vi "Display Info.vi"(7 "Layout ref":refnum<vi>, 8 "error in (no error)":errorcluster, 9 "Modify (F) /Add [T]":bool, 10 "Names in use":string[](array[string])=["PB", "Feet"], 11 "PTS-via-PB in":refnum<class "PTS-via-PB.lvclass">) -> (0 "error out":errorcluster, 1 "Names in use out":string[](array[string]), 2 "Changes Made?":bool, 3 "PTS-via-PB out":refnum<class "PTS-via-PB.lvclass">)   [LabVIEW 2013, in "PTS-via-PB.lvclass"]
uses:
  PTS-via-PB.lvclass
  ColumnVIs/Column/Column.lvclass
  TypeDefs/ColumnAppearCluster.ctl
panel:
  in  "Freq Col":T1={"Column Name"="RF Freq.", "Width"=30, "Bkgd"=[16448250], "Text"=[0]}
  in  "Name":string="PTS"
  in  "Device Description":string
  in  "SpinAPI Path":path=path "C:/SpinCore/SpinAPI/dll/spinapi.dll"
  in  "Board Num.":i32=1 max=256 step=1
  in  "Trig.\nLine":i32=23 max=256 step=1
  in  "Cancel":bool
  in  "Done":bool
  out "Names in use out":string[](array[string])
  out "Cols":refnum<class "Column.lvclass">[](array[class])
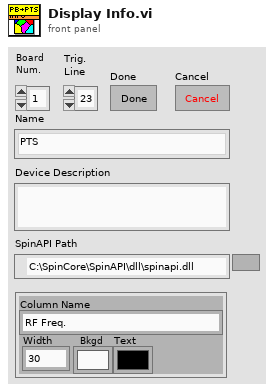
[diagram p1: front panel]
types:
  T1 = typedef "ColumnAppearCluster.ctl" = cluster{"Column Name":string, "Width":u32, "Bkgd":u32[], "Text":u32[]}
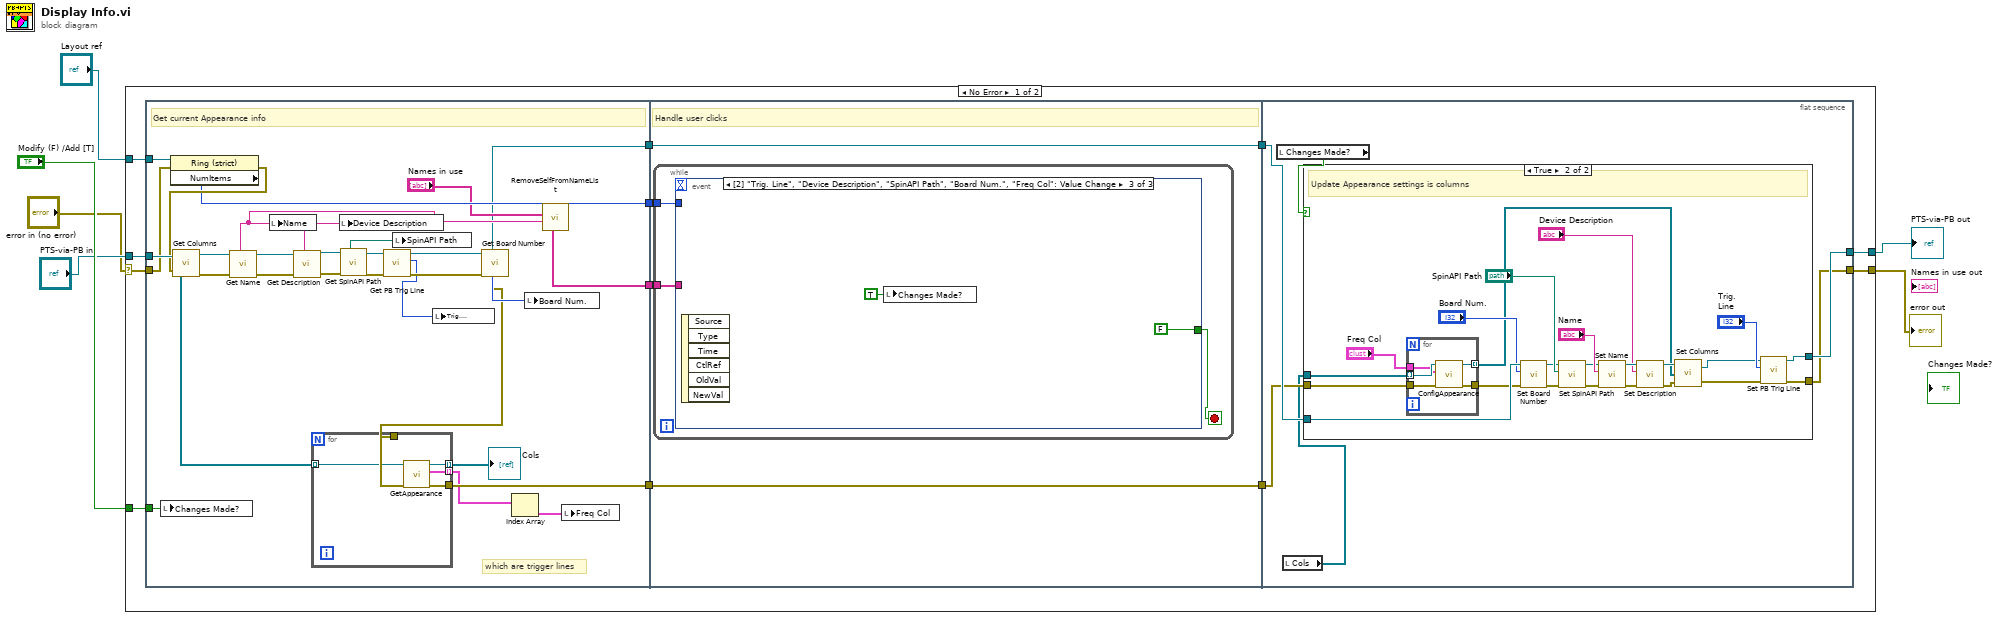
[diagram p0: block diagram]
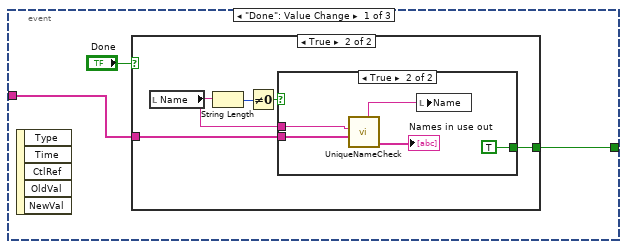
[diagram p2: hidden frame]
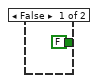
[diagram p3: hidden frame]
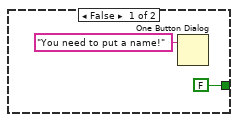
[diagram p4: hidden frame]
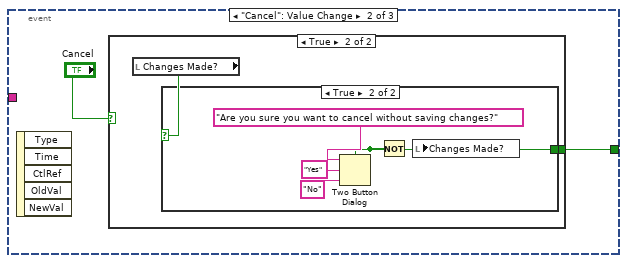
[diagram p5: hidden frame]
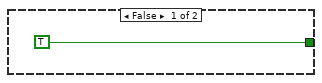
[diagram p7: hidden frame]
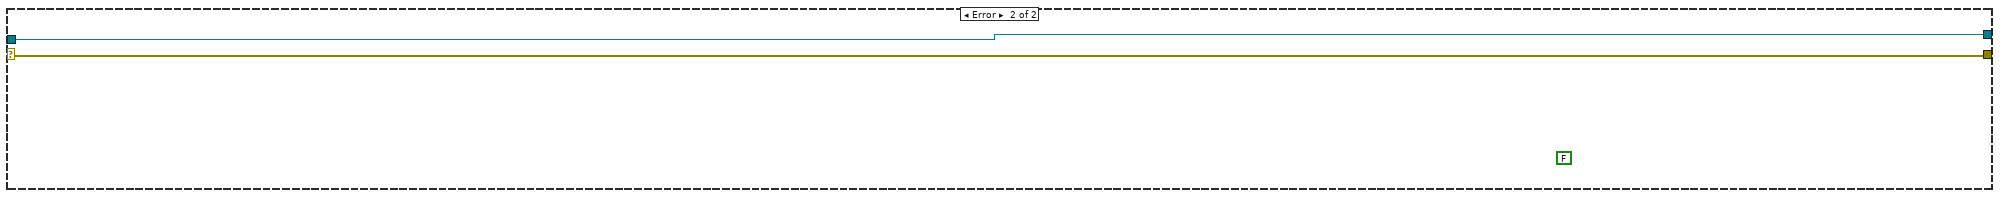
[diagram p9: hidden frame]
diagram:
  n1 = case shown="No Error" "error in (no error)" {
    selector: "error in (no error)" -> [w11 w126]
    tunnel: [w13 w127] -> w2
    tunnel: "PTS-via-PB in" -> [w18 w127]
    tunnel: [w12 w126] -> w1
    tunnel: "Layout ref" -> [w10 _]
    tunnel: "Modify (F) /Add [T]" -> [w8 _]
    frame No Error {
      n2 = flat-sequence {
        tunnel: w18 -> [w46]
        tunnel: [w19] -> w17
        tunnel: [w42] -> w15
        tunnel: w11 -> [w39]
        tunnel: w10 -> [w40]
        tunnel: [w37] -> w9
        tunnel: w8 -> [w36]
        tunnel: [w34] -> w7
        tunnel: w17 -> [w57]
        tunnel: [w57] -> w16
        tunnel: w15 -> [w56]
        tunnel: [w56] -> w14
        tunnel: w9 -> [w55]
        tunnel: w7 -> [w54]
        tunnel: w16 -> [w94]
        tunnel: w14 -> [w91]
        tunnel: [w93] -> w13
        tunnel: [w92] -> w12
        frame #0 {
          # "which are trigger lines"
          # "Get current Appearance info"
          n3 = local write "Changes Made?"(w36) -> ()
          n4 = property class="Ring (strict)"(reference=w40, error in=w39) -> (error out=w38:errorcluster, "NumItems"=w37:u32)  [unwired: 1 out]
          n5 = call-dynamic "Get Columns.vi"("Device in"=w46, "error in (no error)"=w38) -> ("Device out"=w44:refnum<class "PTS-via-PB.lvclass">, "Columns"=w29:refnum<class "Column.lvclass">[], "error out"=w43:errorcluster)
          n6 = call-dynamic "Get Name.vi"("error in (no error)"=w43, "Device in"=w44) -> ("error out"=w45:errorcluster, "Name"=w35:string, "Device out"=w48:refnum<class "PTS-via-PB.lvclass">)  [unwired: 7 in]
          n7 = local write "Name"(w35) -> ()
          n8 = call-dynamic "Get Description.vi"("error in (no error)"=w45, "Device in"=w48) -> ("error out"=w32:errorcluster, "Device Description"=w47:string, "Device out"=w33:refnum<class "PTS-via-PB.lvclass">)  [unwired: 7 in]
          n9 = local write "Device Description"(w47) -> ()
          n10 = call-dynamic "Get SpinAPI Path.vi"("error in (no error)"=w32, "Pulseblaster in"=w33) -> ("error out"=w25:errorcluster, "SpinAPI Path"=w30:path, "Pulseblaster out"=w26:refnum<class "PTS-via-PB.lvclass">)  [unwired: 7 in]
          n11 = call-dynamic "Get PB Trig Line.vi"("error in (no error)"=w25, "Device in"=w26) -> ("error out"=w23:errorcluster, "PB Trigger Line"=w22:u16, "Device out"=w24:refnum<class "PTS-via-PB.lvclass">)  [unwired: 7 in]
          n12 = local write "SpinAPI Path"(w30) -> ()
          n13 = local write "Trig.\nLine"(w22) -> ()
          n14 = call-dynamic "Get Board Number.vi"("error in (no error)"=w23, "Pulseblaster in"=w24) -> ("error out"=w28:errorcluster, "Board Number"=w31:i32, "Pulseblaster out"=w19:refnum<class "PTS-via-PB.lvclass">)  [unwired: 7 in]
          n15 = for {
            tunnel: w29 -> [w49] mode=indexing
            tunnel: [w53] -> w27 mode=indexing
            tunnel: [w52] -> w42
            tunnel: w28 -> [w51]
            tunnel: [w50] -> w20 mode=indexing
            n16 = call "GetAppearance.vi"("error in (no error)"=w51, "Column in"=w49) -> ("error out"=w52:errorcluster, "Column Appearance"=w53:T1, "Column out"=w50:refnum<class "Column.lvclass">)  [unwired: 7 in]
          }
          "Cols" <- w20
          n17 = Index Array(array=w27) -> (element=w41:T1)  [unwired: 1 in]
          n18 = local write "Board Num."(w31) -> ()
          n19 = call "RemoveSelfFromNameList.vi"("self Name"=w35, "Names in use"="Names in use") -> ("Reserved Names"=w34:string[])  [unwired: 9 in]
          n20 = local write "Freq Col"(w41) -> ()
        }
        frame #1 {
          # "Handle user clicks"
          n21 = while {
            tunnel: w55 -> [w59]
            tunnel: w54 -> [w58]
            stop <- w60 stop-if-true
            n22 = event shown="[2] \"Trig. Line\", \"Device Description\", \"SpinAPI Path\", \"Board Num.\", \"Freq Col\": Value Change" {
              selector: _ -> [_ _ _]
              dyn-events: _ -> [_ _ _]
              timeout: _ -> [_ _ _]
              tunnel: [w62 w78 FALSE ("T button?")] -> w60
              tunnel: w59 -> [_ _ _]
              tunnel: w58 -> [w61 _ _]
              event "Done": Value Change {
                n23 = event-data() -> ()  [unwired: 1 in, 5 out]
                n24 = case shown="True" "Done" {
                  tunnel: [FALSE w67] -> w62
                  tunnel: w61 -> [_ w65]
                  frame False {
                  }
                  frame True {
                    n25 = local read "Name"() -> (w66:string)
                    n26 = String Length(string=w66) -> (length=w69:i32)
                    n27 = Not Equal To 0?(x=w69) -> (x != 0?=w68:bool)
                    n28 = case shown="True" w68 {
                      tunnel: [FALSE TRUE] -> w67
                      tunnel: w66 -> [_ w75]
                      tunnel: w65 -> [_ w73]
                      frame False {
                        n29 = One Button Dialog(message="You need to put a name!") -> ()  [unwired: 1 in, 1 out]
                      }
                      frame True {
                        n30 = call "UniqueNameCheck.vi"("Names in use"=w73, "Device Name"=w75) -> ("Names in use out"=→"Names in use out":string[], "Unique name"=w74:string)  [unwired: 8 in]
                        n31 = local write "Name"(w74) -> ()
                      }
                    }
                  }
                }
              }
              event "Cancel": Value Change {
                n32 = event-data() -> ()  [unwired: 1 in, 5 out]
                n33 = case shown="True" "Cancel" {
                  selector: "Cancel" -> [w79 _]
                  tunnel: [w79 w81] -> w78
                  frame False {
                  }
                  frame True {
                    n34 = local read "Changes Made?"() -> (w80:bool)
                    n35 = case shown="True" w80 {
                      tunnel: [TRUE w84] -> w81
                      frame False {
                      }
                      frame True {
                        n36 = Two Button Dialog(message="Are you sure you want to cancel without saving changes?", 1:"No", 2:"Yes") -> (T button?=w84:bool)
                        n37 = Not(x=w84) -> (.not. x?=w83:bool)
                        n38 = local write "Changes Made?"(w83) -> ()
                      }
                    }
                  }
                }
              }
              event "Trig.\nLine", "Device Description", "SpinAPI Path", "Board Num.": Value Change {
                n39 = event-data() -> ()  [unwired: 1 in, 6 out]
                n40 = local write "Changes Made?"(TRUE) -> ()
              }
            }
          }
        }
        frame #2 {
          n41 = local read "Changes Made?"() -> (w95:bool)
          n42 = local read "Cols"() -> (w90:refnum<class "Column.lvclass">[])
          n43 = case shown="True" w95 {
            tunnel: w94 -> [w97 w109]
            tunnel: [w96 w101] -> w92
            tunnel: [w97 w102] -> w93
            tunnel: w91 -> [w96 w115]
            tunnel: w90 -> [_ w114]
            frame False {
            }
            frame True {
              # "Update Appearance settings is columns"
              n44 = for {
                tunnel: [w125] -> w105 mode=indexing
                tunnel: [w124] -> w104
                tunnel: w114 -> [w123] mode=indexing
                tunnel: w115 -> [w122]
                tunnel: "Freq Col" -> [w121]
                n45 = call "ConfigAppearance.vi"("error in (no error)"=w122, "Column Appearance"=w121, "Column in"=w123) -> ("error out"=w124:errorcluster, "Column out"=w125:refnum<class "Column.lvclass">)  [unwired: 7 in]
              }
              n46 = call-dynamic "Set Board Number.vi"("error in (no error)"=w104, "Board Number"="Board Num.", "Pulseblaster in"=w109) -> ("error out"=w110:errorcluster, "Pulseblaster out"=w108:refnum<class "PTS-via-PB.lvclass">)  [unwired: 7 in]
              n47 = call-dynamic "Set SpinAPI Path.vi"("error in (no error)"=w110, "SpinAPI Path"="SpinAPI Path", "Pulseblaster in"=w108) -> ("error out"=w111:errorcluster, "Pulseblaster out"=w107:refnum<class "PTS-via-PB.lvclass">)  [unwired: 7 in]
              n48 = call-dynamic "Set Name.vi"("error in (no error)"=w111, "Name"="Name", "Device in"=w107) -> ("error out"=w120:errorcluster, "Device out"=w119:refnum<class "PTS-via-PB.lvclass">)  [unwired: 7 in]
              n49 = call-dynamic "Set Description.vi"("error in (no error)"=w120, "Device Description"="Device Description", "Device in"=w119) -> ("error out"=w113:errorcluster, "Device out"=w118:refnum<class "PTS-via-PB.lvclass">)  [unwired: 7 in]
              n50 = call-dynamic "Set Columns.vi"("error in (no error)"=w113, "Columns in"=w105, "Pulseblaster in"=w118) -> ("error out"=w103:errorcluster, "Pulseblaster out"=w98:refnum<class "PTS-via-PB.lvclass">)  [unwired: 1 in]
              n51 = call-dynamic "Set PB Trig Line.vi"("error in (no error)"=w103, "PB Trigger Line"="Trig.\nLine", "Device in"=w98) -> ("error out"=w101:errorcluster, "Device out"=w102:refnum<class "PTS-via-PB.lvclass">)  [unwired: 7 in]
            }
          }
        }
      }
    }
    frame Error {
      (unwired) FALSE
    }
  }
  "error out" <- w1
  "PTS-via-PB out" <- w2
